vi "ex7.vi"() -> ()   [LabVIEW 2022 SP3]
panel:
  out "valid?":bool
  in  "password":string
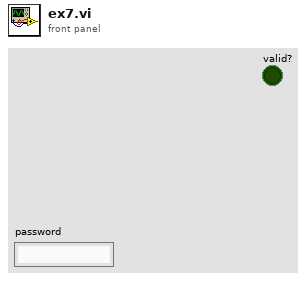
[diagram p1: front panel]
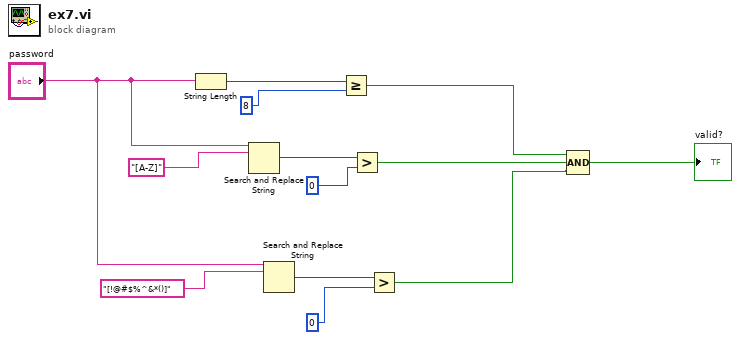
[diagram p0: block diagram]
diagram:
  n1 = String Length(string="password") -> (length=w12:i32)
  n2 = Search and Replace String(input string="password", search string="[A-Z]") -> (number of replacements=w9:i32)  [unwired: 6 in, 3 out]
  n3 = Search and Replace String(input string="password", search string="[!@#$%^&*()]") -> (number of replacements=w5:i32)  [unwired: 6 in, 3 out]
  n4 = Greater Or Equal?(x=w12, y=8) -> (x >= y?=w3:bool)
  n5 = Greater?(x=w9, y=0) -> (0:w2:bool)
  n6 = Greater?(x=w5, y=0) -> (0:w1:bool)
  n7 = Compound Arithmetic op=AND(w3, w2, w1) -> (→"valid?":bool)
